vi "GSI-HVSwitch2.get data to modify.vi"(0 "i ref in":refnum<vi>, 3 "ms timeout (10000)":i32=10000, 5 "error in (no error)":errorcluster) -> (14 "i ref out":refnum<vi>, 16 "i attribute":T1={"SDEX VISA Cluster"={"VISA resource name"="", "HEX address"=0, "VISA Timeout Value (1000 ms)"=1000, "Lock Timeout (1000 ms)"=1000, "semaphore"=refnum, "Baud rate"=0, "revision"=enum."unknown", "deviceInfo"=""}, "SetVoltage SW0"=0.0, "SetVoltage SW1"=0.0, "ActTempAmp"=0.0, "ActTempPS1"=0.0, "ActTempPS2"=0.0, "mode"=enum."unknown", "interfaceInitialized"=FALSE, "serviceIDs"={"nomVoltage0ID"=0, "nomVoltage1ID"=0, "actTempAmpID"=0, "actTempPS1ID"=0, "actTempPS2ID"=0, "modeID"=0}, "usedChannels"=0} {"SDEX VISA Cluster"."HEX address" format="%.0x"}, 17 "timed out":bool, 19 "error out":errorcluster)   [LabVIEW 2014, in "GSI-HVSwitch2.lvlib"]
doc: "Reads the attribute data of the object after the access to the data has been locked by the \"acquire\" method. If the attribute data has been locked already, this methods waits until the attribute data is unlocked or there is a timeout.\n\nThe attribute data must be unlocked using the methods \"release\" or \"set modified data\".\n\nLicense Agreement for this software:\n\nCopyright (C)\nGesellschaft für Schwerionenforschung, GSI\nPlanckstr. 1\n64291 Darmstadt\nGermany\n\nContact: D.Beck@gsi.de \n\nThis program is free software; you can redistribute it and/or modify it under the terms of the GNU General Public License as published by the Free Software Foundation; either version 2 of the license, or (at your option) any later version.\n\nThis program is distributed in the hope that it will be useful, but WITHOUT ANY WARRANTY; without even the implied warranty of MERCHANTABILITY or FITNESS FOR A PARTICULAR PURPOSE. See the GNU General License for more details (http://www.gnu.org).\n\nGesellschaft für Schwerionenforschung, GSI\nPlanckstr. 1, 64291 Darmstadt, Germany\nFor all questions and ideas contact: M.Richter@gsi.de, H.Brand@gsi.de or D.Beck@gsi.de.\nLast update: 17-JUN-2004"
uses:
  GSI-HVSwitch2.lvlib
  GSI-HVSwitch2.i attribute.ctl
  instr.lib/SDEX/SDEX.VISA Control.ctl
  instr.lib/SDEX/SDEX.revisionType.ctl
  GSI-HVSwitch2.mode.ctl
  CS_Core/CSObj/CSObj.lvlib
  instr.lib/SDEX/SDEXDriver.lvlib
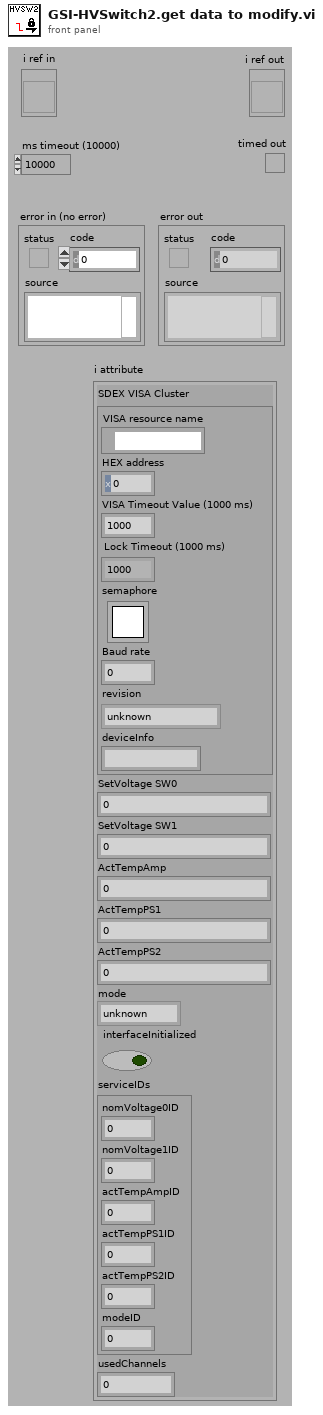
[diagram p1: front panel]
types:
  T1 = typedef "GSI-HVSwitch2.lvlib/GSI-HVSwitch2.i attribute.ctl" = cluster{"SDEX VISA Cluster":T2, "SetVoltage SW0":dbl, "SetVoltage SW1":dbl, "ActTempAmp":dbl, "ActTempPS1":dbl, "ActTempPS2":dbl, "mode":T5, "interfaceInitialized":bool, "serviceIDs":cluster{"nomVoltage0ID":i32, "nomVoltage1ID":i32, "actTempAmpID":i32, "actTempPS1ID":i32, "actTempPS2ID":i32, "modeID":i32}, "usedChannels":i32}
  T2 = typedef "SDEXDriver.lvlib/SDEX.VISA Control.ctl" = cluster{"VISA resource name":refnum<visa-resource-name>, "HEX address":u16, "VISA Timeout Value (1000 ms)":u32, "Lock Timeout (1000 ms)":u32, "semaphore":T3, "Baud rate":u32, "revision":T4, "deviceInfo":string}
  T3 = typedef "Semaphore RefNum" = refnum<k1>
  T4 = typedef "SDEXDriver.lvlib/SDEX.revisionType.ctl" = enum16{"unknown", "hvamp3", "hvswi1", "htrp0", "WDG0"}
  T5 = typedef "GSI-HVSwitch2.lvlib/GSI-HVSwitch2.mode.ctl" = enum16{"unknown", "switch", "stepper"}
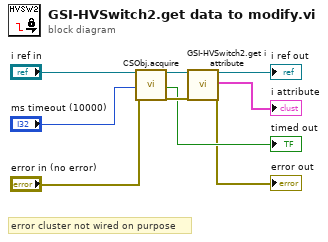
[diagram p0: block diagram]
diagram:
  # "error cluster not wired on purpose"
  n1 = call "CSObj.acquire.vi"("i ref in"="i ref in", "ms timeout (10000)"="ms timeout (10000)", "error in (no error)"="error in (no error)") -> ("i ref out"=w8:refnum<vi>, "timed out"=→"timed out":bool, "error out"=w5:errorcluster)  [unwired: 14 in]
  n2 = call "GSI-HVSwitch2.get i attribute.vi"("i ref in"=w8, "error in (no error)"=w5) -> ("i ref out"=→"i ref out":refnum<vi>, "i attribute"=→"i attribute":T1, "error out"=→"error out":errorcluster)  [unwired: 15 in]
